vi "ReadTemperature.vi"(8 "error in (no error)":errorcluster, 11 "dvotTTPathPoint in":refnum<class "dvotTTPathPoint.lvclass">) -> (0 "error out":errorcluster, 2 "temperature":dbl, 3 "dvotTTPathPoint out":refnum<class "dvotTTPathPoint.lvclass">)   [LabVIEW 2012, in "dvotTTPathPoint.lvclass"]
uses:
  dvotTTPathPoint.lvclass
  dvotTTPathPoint.lvclass/dvotTTPathPoint.ctl
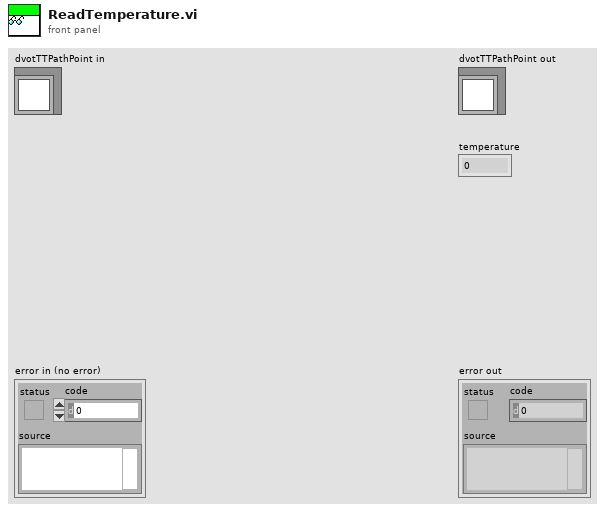
[diagram p1: front panel]
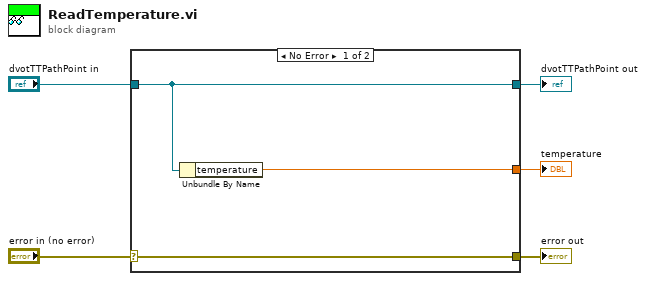
[diagram p0: block diagram]
diagram:
  n1 = case shown="No Error" "error in (no error)" {
    selector: "error in (no error)" -> [w8 w9]
    tunnel: [w8 w9] -> w4
    tunnel: [w7 w10] -> w2
    tunnel: "dvotTTPathPoint in" -> [w7 w10]
    tunnel: [w6 _] -> w1
    frame No Error {
      n2 = Unbundle By Name(w7) -> ("temperature"=w6:dbl)
    }
    frame Error {
    }
  }
  "error out" <- w4
  "dvotTTPathPoint out" <- w2
  "temperature" <- w1
